vi "MotorOutput_Simulation_Global.vi"(0 "menu":enum16{"set", "get", "delete"}(ring)=enum."get", 7 "PWM Channel":T1=enum."PWM 1", 9 "Output Set":dbl format="%#.4f", 11 "error in (no error)":errorcluster) -> (10 "Output Get":dbl format="%#.4f", 15 "error out":errorcluster)   [LabVIEW 2017]
doc: "This is used to set and get the last motor output values. This is needed for simulation, since we cannot read these values from the hardware.\n\nThis software is licensed. Open the labview\\readme\\WPI Robotics Library Open Source License.txt file for more information."
uses:
  <vilib>/Rock Robotics/SystemInterfaces/DIO/FPGA_DIOPWMChannel.ctl
panel:
  out "Array":dbl[](array[numeric]) format="%#.4f"
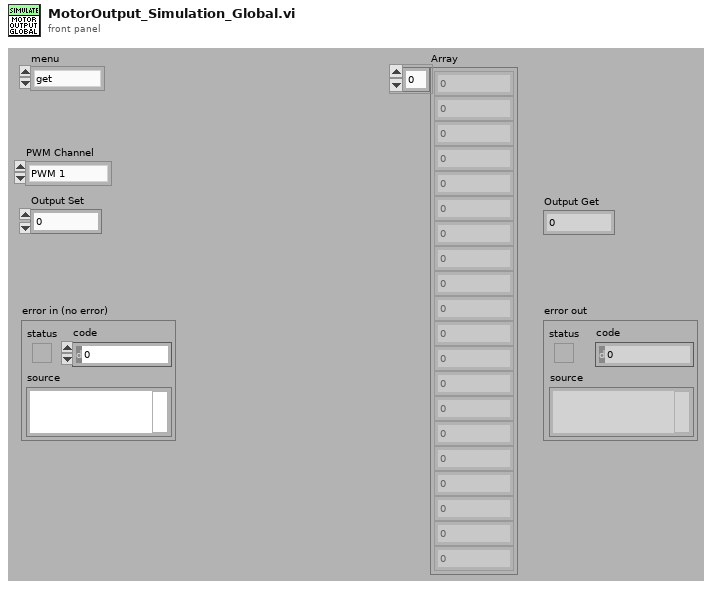
[diagram p1: front panel]
types:
  T1 = typedef "FPGA_DIOPWMChannel.ctl" = enum8{"PWM 0", "PWM 1", "PWM 2", "PWM 3", "PWM 4", "PWM 5", "PWM 6", "PWM 7", "PWM 8", "PWM 9", "PWM MXP 0", "PWM MXP 1", "PWM MXP 2", "PWM MXP 3", "PWM MXP 4", "PWM MXP 5", "PWM MXP 6", "PWM MXP 7", "PWM MXP 8", "PWM MXP 9", "Invalid"}
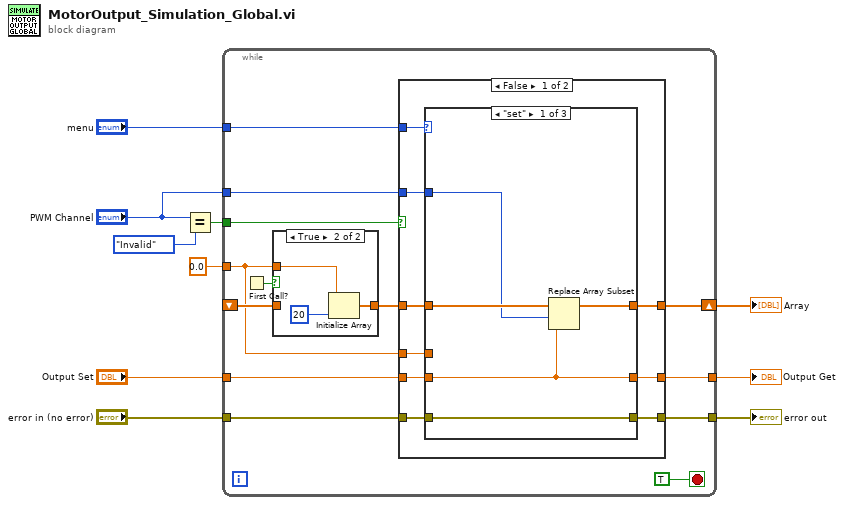
[diagram p0: block diagram]
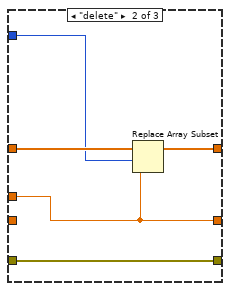
[diagram p2: hidden frame]
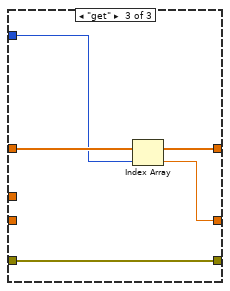
[diagram p3: hidden frame]
diagram:
  n1 = Equal?(x="PWM Channel", y=FPGA_DIOPWMChannel."Invalid" ("PWM Channel")) -> (x = y?=w7:bool)
  n2 = while {
    tunnel: "Output Set" -> [w23]
    tunnel: "error in (no error)" -> [w19]
    shift-right: [w22] -> w6
    shift-left: _ -> [w14]
    tunnel: [w21] -> w2
    tunnel: "menu" -> [w20]
    tunnel: [w18] -> w9
    tunnel: "PWM Channel" -> [w13]
    tunnel: w7 -> [w12]
    tunnel: 0.0 ("Output") -> [w11]
    stop <- TRUE stop-if-true
    n3 = First Call?() -> (First Call?: T/F=w16:bool)
    n4 = case shown="True" w16 {
      tunnel: [w50 w52] -> w15
      tunnel: w14 -> [w50 _]
      tunnel: w11 -> [_ w51]
      frame False {
      }
      frame True {
        n5 = Initialize Array(w51, 20 ("dimension size")) -> (w52:dbl[])
      }
    }
    n6 = case shown="False" w12 {
      tunnel: w23 -> [w32 _]
      tunnel: [w31 w49] -> w22
      tunnel: [w30 w47] -> w21
      tunnel: w20 -> [w29 _]
      tunnel: w19 -> [w28 w48]
      tunnel: [w27 w48] -> w18
      tunnel: w15 -> [w26 w49]
      tunnel: w13 -> [w25 _]
      tunnel: w11 -> [w24 w47]
      frame False {
        n7 = case shown="\"set\"" w29 {
          tunnel: w32 -> [w35 _ _]
          tunnel: [w36 w41 w46] -> w31
          tunnel: w26 -> [w37 w42 w46]
          tunnel: [w35 w38 w45] -> w30
          tunnel: [w34 w40 w44] -> w27
          tunnel: w28 -> [w34 w40 w44]
          tunnel: w25 -> [w33 w39 w43]
          tunnel: w24 -> [_ w38 _]
          frame "set" {
            n8 = Replace Array Subset(array=w37, new element=w35, index=w33) -> (w36:dbl[])
          }
          frame "delete" {
            n9 = Replace Array Subset(array=w42, new element=w38, index=w39) -> (w41:dbl[])
          }
          frame "get" {
            n10 = Index Array(array=w46, index=w43) -> (element=w45:dbl)
          }
        }
      }
      frame True {
        # "Do nothing if PWM channel is Invalid."
      }
    }
  }
  "error out" <- w9
  "Array" <- w6
  "Output Get" <- w2
